vi "SetCommand.vi"(0 "Simulated Device in":refnum<class "Simulated Device.lvclass">, 1 "Device Code":T2, 5 "Parameter 1":string, 7 "Parameter 2":string, 9 "Parameter 3":string, 11 "error in (no error)":errorcluster, 12 "Command Code":T1) -> (4 "Simulated Device out":refnum<class "Simulated Device.lvclass">, 6 "Command":string, 15 "error out":errorcluster)   [LabVIEW 2020, in "Simulated Device.lvclass"]
doc: "It creats a command concatenating the given parameters. According to the device, it would send the command through the corresponding communication bus."
uses:
  Simulated Device.lvclass
  Controls/Device Code.ctl
  Controls/Device Command Code.ctl
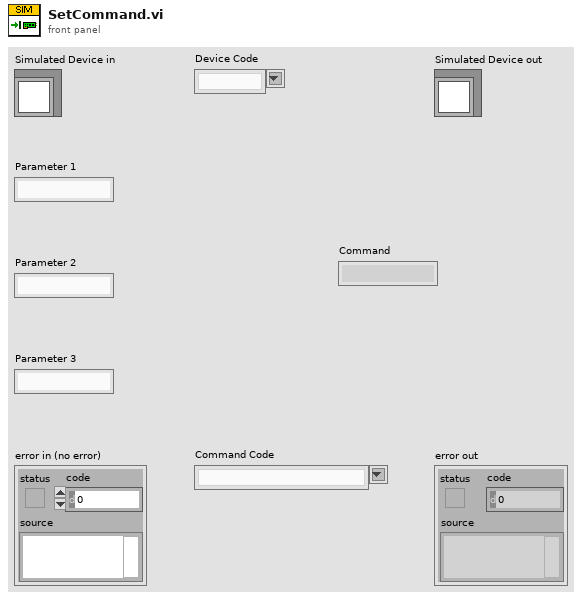
[diagram p1: front panel]
types:
  T1 = typedef "Device Command Code.ctl" = string
  T2 = typedef "Device Code.ctl" = string
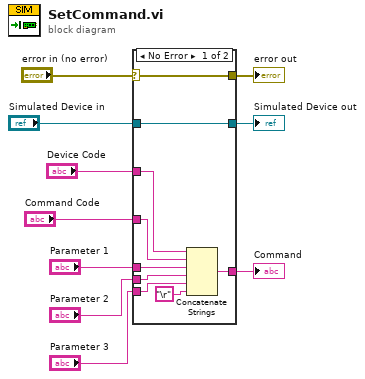
[diagram p0: block diagram]
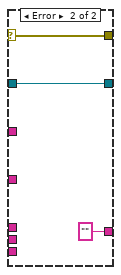
[diagram p2: hidden frame]
diagram:
  n1 = case shown="No Error" "error in (no error)" {
    selector: "error in (no error)" -> [w13 w22]
    tunnel: "Device Code" -> [w19 _]
    tunnel: "Command Code" -> [w18 _]
    tunnel: "Parameter 1" -> [w17 _]
    tunnel: "Parameter 2" -> [w16 _]
    tunnel: "Parameter 3" -> [w15 _]
    tunnel: "Simulated Device in" -> [w14 w21]
    tunnel: [w14 w21] -> w3
    tunnel: [w13 w22] -> w1
    tunnel: [w11 ""] -> w2
    frame No Error {
      n2 = Concatenate Strings(w19, w18, w17, w16, w15, "\r") -> (w11:string)
    }
    frame Error {
    }
  }
  "error out" <- w1
  "Simulated Device out" <- w3
  "Command" <- w2
